vi "SDT_GenerateBHFileBlockHeaderDecayCurves.vi"(7 "ModuleNo":u32, 10 "BlockLengths":i32[](array[numeric]), 11 "data_block_offs":i32) -> (2 "BHFileBlockHeaders":T1[](array[typedef]), 3 "BlockHeaderLength":i32)   [LabVIEW 2017]
doc: "This VI is a SubVI to SDT_WriteFile.vi. It populates the clusters BHFileBlockHeader ready to be written to file. \nFor a description of the *.sdt file format see: SPC_data_file_structure.h\n\ninfo@becker-hickl.com"
uses:
  SPC_Wrappers/SPC_Controls/BHFileBlockHeader.ctl
  SPC_Wrappers/SPC_Controls/BlockType_Contents.ctl
  SPC_Wrappers/SPC_Controls/BlockType_DataType.ctl
  SPC_Wrappers/SPC_Controls/BlockType_CreationMode.ctl
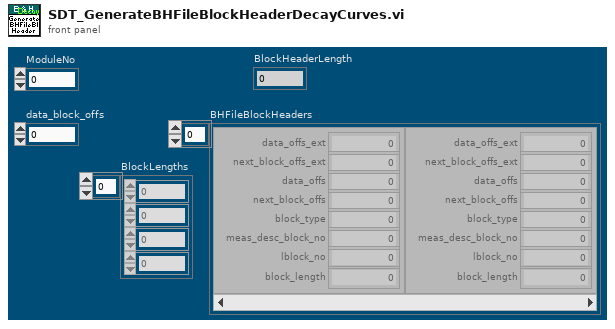
[diagram p1: front panel]
types:
  T1 = typedef "BHFileBlockHeader.ctl" = cluster{"data_offs_ext":u8, "next_block_offs_ext":u8, "data_offs":u32, "next_block_offs":u32, "block_type":u16, "meas_desc_block_no":i16, "lblock_no":u32, "block_length":u32}
  T2 = typedef "BlockType_DataType.ctl" = u16
  T3 = typedef "BlockType_Contents.ctl" = u16
  T4 = enum16{"big-endian, network order", "native, host order", "little-endian"}
  T5 = typedef "BlockType_CreationMode.ctl" = u16
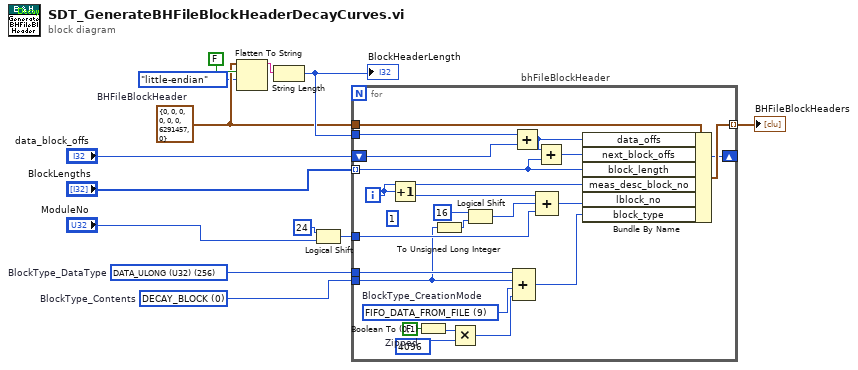
[diagram p0: block diagram]
diagram:
  w5 = T1 {"data_offs_ext"=0, "next_block_offs_ext"=0, "data_offs"=0, "next_block_offs"=0, "block_type"=0, "meas_desc_block_no"=0, "lblock_no"=6291457, "block_length"=0}  # BHFileBlockHeader
  w2 = T2 256 items=["DATA_USHORT (U16)"=0, "DATA_ULONG (U32)"=256, "DATA_DBL (DBL64)"=512]  # BlockType_DataType
  w1 = T3 0 items=["DECAY_BLOCK"=0, "PAGE_BLOCK"=16, "FCS_BLOCK"=32, "FIDA_BLOCK"=48, "FILDA_BLOCK"=64, "MCS_BLOCK"=80, "IMG_BLOCK"=96, "MCST_BLOCK"=112, "IMG_MCS_BLOCK"=128, "MOM_BLOCK"=144, "IMG_INT_BLOCK"=160, "IMG_WF_BLOCK"=176, "IMG_LIFE_BLOCK"=192]  # BlockType_Contents
  n1 = Flatten To String(anything=w5, prepend array or string size? (T)=FALSE, byte order (0:big-endian, network order)=T4."little-endian") -> (data string=w3:string)  [unwired: 1 in, 2 out]
  n2 = String Length(string=w3) -> (length=w7:i32)
  "BlockHeaderLength" <- w7
  n3 = Logical Shift(y=i16 24, x="ModuleNo") -> (x << y=w9:u32)
  n4 = for "bhFileBlockHeader" {
    tunnel: w7 -> [w33]
    tunnel: w2 -> [w20]
    tunnel: w1 -> [w19]
    tunnel: w5 -> [w34]
    tunnel: [w35] -> w11 mode=indexing
    tunnel: "BlockLengths" -> [w16] mode=indexing
    shift-right: [w26] -> _
    shift-left: "data_block_offs" -> [w25]
    tunnel: w9 -> [w21]
    i -> [w15]
    (unwired) 1
    w31 = FALSE  # Zipped
    w32 = T5 9 items=["NOT_USED"=0, "MEAS_DATA"=1, "FLOW_DATA"=2, "MEAS_DATA_FROM_FILE"=3, "CALC_DATA"=4, "SIM_DATA"=5, "FIFO_DATA"=8, "FIFO_DATA_FROM_FILE"=9, "MOM_DATA"=10, "MOM_DATA_FROM_FILE"=11]  # BlockType_CreationMode
    n5 = Increment(x=w15) -> (x+1=w14:i32)
    n6 = Boolean To (0,1)(Boolean=w31) -> (0, 1=w30:i16)
    n7 = To Unsigned Long Integer(number=w19) -> (unsigned 32bit integer=w18:u32)
    n8 = Multiply(x=w30, y=u16 4096) -> (x*y=w28:u16)
    n9 = Logical Shift(y=u16 16, x=w18) -> (x << y=w24:u32)
    n10 = Add(x=w33, y=w25) -> (x+y=w27:i32)
    n11 = Compound Arithmetic op=unknown(w20, w19, w32, w28) -> (w17:T2)
    n12 = Add(x=w27, y=w16) -> (x+y=w26:i32)
    n13 = Compound Arithmetic op=ADD(w14, w24, w21) -> (w23:u32)
    n14 = Bundle By Name(cluster=w34, "data_offs"=w27, "next_block_offs"=w26, "block_length"=w16, "meas_desc_block_no"=w15, "lblock_no"=w23, "block_type"=w17) -> (w35:T1)
  }
  "BHFileBlockHeaders" <- w11
